vi "DC Attenuation Unflatten Test Parameters.vi"(9 "error in (no error)":errorcluster, 10 "Parameter String":string) -> (1 "error out":errorcluster, 2 "DC Attenuation Test Parameters":T2={"Stimulus"={"Use Instrument"=FALSE, "Normalize"=FALSE, "Blank Screen"=FALSE, "Measurement Type"=enum."Diode", "Range"=enum."Auto", "Resolution"=enum."Auto"}, "Measurement"={"Topology"=enum."PI-Network", "Lock Topology"=FALSE, "ATTN Calc"=enum."Power", "Zo"=50.0}, "Limits"=[], "Normalization"={"Normalized?"=FALSE, "Rab Value"=0.0, "Rac Value"=0.0, "Rbc Value"=0.0}}, 5 "Test Version":string)   [LabVIEW 2011]
uses:
  TypeDefs/DCA Test Parameters.ctl
  TypeDefs/DCA Stimulus Parameters.ctl
  TypeDefs/DCA Measurement Cluster.ctl
  TypeDefs/DCA Topology.ctl
  TypeDefs/DCA Attenuation Calculation.ctl
  TypeDefs/DCA Limit.ctl
  TypeDefs/DCA Limit Quantity.ctl
  TypeDefs/DCA Limit Comparison.ctl
  TypeDefs/DCA Limit Operation.ctl
  Test Referential Limit.ctl
  TypeDefs/DCA Calibration State.ctl
  Test Return Parameter.ctl
  TypeDefs/DCA Test Parameters v1.0-1.1.ctl
  TypeDefs/DCA Test Parameters v1.2.ctl
  TypeDefs/DCA Test Parameters v1.3-1.4.ctl
  TypeDefs/DCA Test Parameters v1.5.ctl
  TypeDefs/DCA Test Parameters v1.6-1.7.ctl
  TypeDefs/DCA Test Parameters v1.8.ctl
  TypeDefs/DCA Test Parameters v1.9.ctl
panel:
  in  "Return Parameter":T1
  out "Parameter Variant":variant
  in  "Required Instruments":string[](array[string])=["DMM", "SWI"]
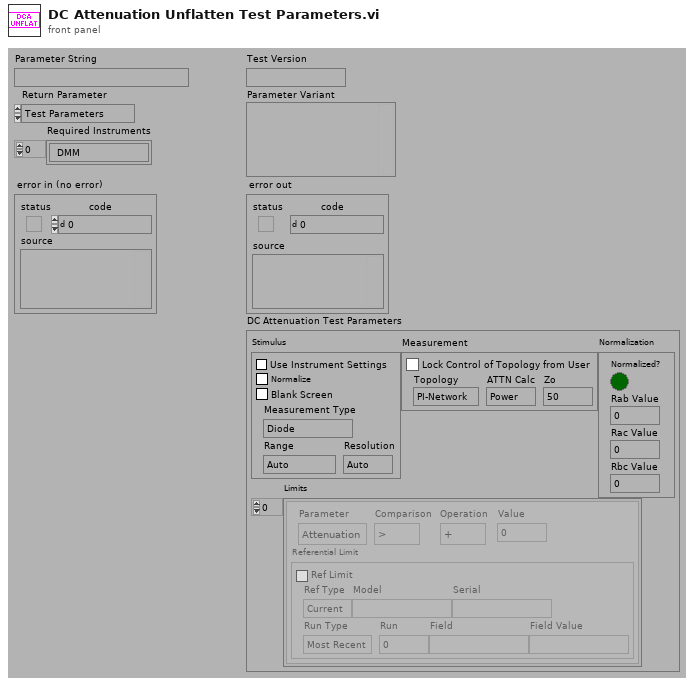
[diagram p1: front panel]
types:
  T1 = typedef "Test Return Parameter.ctl" = enum16{"Test Parameters", "Required Instruments", "Datasheets", "QuickMode"}
  T2 = typedef "DCA Test Parameters.ctl" = cluster{"Stimulus":T3, "Measurement":T4, "Limits":T7[], "Normalization":T12}
  T3 = typedef "DCA Stimulus Parameters.ctl" = cluster{"Use Instrument":bool, "Normalize":bool, "Blank Screen":bool, "Measurement Type":enum16{"Voltage DC", "Voltage DC Ratio", "Voltage AC", "Current DC", "Current AC", "Resistance", "Fresistance", "Frequency", "Period", "Continuity", "Diode"}, "Range":enum16{"Auto", "Minimum", "Maximum", "100", "1,000", "10,000", "100,000", "1,000,000", "10,000,000", "100,000,000"}, "Resolution":enum16{"Auto", "4 1/2", "5 1/2", "6 1/2"}}
  T4 = typedef "DCA Measurement Cluster.ctl" = cluster{"Topology":T5, "Lock Topology":bool, "ATTN Calc":T6, "Zo":dbl}
  T5 = typedef "DCA Topology.ctl" = enum32{"PI-Network", "T-Network"}
  T6 = typedef "DCA Attenuation Calculation.ctl" = enum32{"Power", "Voltage"}
  T7 = typedef "DCA Limit.ctl" = cluster{"Parameter":T8, "Comparison":T9, "Operation":T10, "Value":dbl, "Referential Limit":T11}
  T8 = typedef "DCA Limit Quantity.ctl" = enum16{"Attenuation", "Zin", "Zout", "R1", "R2", "R3", "Rab", "Rac", "Rbc"}
  T9 = typedef "DCA Limit Comparison.ctl" = enum16{">", ">=", "<", "<="}
  T10 = typedef "DCA Limit Operation.ctl" = enum16{"+", "-"}
  T11 = typedef "Test Referential Limit.ctl" = cluster{"Ref Limit":bool, "Ref Type":enum16{"Current", "Specify"}, "Model":string, "Serial":string, "Run Type":enum16{"Most Recent", "Run #", "Match Field"}, "Run":i32, "Field":string, "Field Value":string}
  T12 = typedef "DCA Calibration State.ctl" = cluster{"Normalized?":bool, "Rab Value":dbl, "Rac Value":dbl, "Rbc Value":dbl}
  T13 = typedef "DCA Test Parameters v1.0-1.1.ctl" = cluster{"Tag":string, "Use Instrument":bool, "Quick Mode":bool, "Topology":enum32{"Pi", "T"}, "Zo":dbl, "Range":u16, "Resolution":u16, "Blank Screen":bool, "Limits":cluster{"Quantity":enum16{"Attenuation", "Zin", "Zout", "R1", "R2", "R3", "Rab", "Rac", "Rbc"}, "Comparison":enum16{">", ">=", "<", "<="}, "Value":dbl}[], "Reports":i32[], "Lock Topology":bool}
  T14 = typedef "DCA Test Parameters v1.2.ctl" = cluster{"Tag":string, "Use Instrument":bool, "Quick Mode":bool, "Topology":enum32{"Pi", "T"}, "Zo":dbl, "Range":u16, "Resolution":u16, "Blank Screen":bool, "Limits":cluster{"Quantity":enum16{"Attenuation", "Zin", "Zout", "R1", "R2", "R3", "Rab", "Rac", "Rbc"}, "Comparison":enum16{">", ">=", "<", "<="}, "Value":dbl}[], "Reports":cluster{"Reports to Generate":i32[], "Print Reports":bool}, "Lock Topology":bool}
  T15 = typedef "DCA Test Parameters v1.3-1.4.ctl" = cluster{"Tag":string, "Use Instrument":bool, "Quick Mode":bool, "Topology":enum32{"Pi", "T"}, "Zo":dbl, "Range":u16, "Resolution":u16, "Blank Screen":bool, "Limits":cluster{"Quantity":enum16{"Attenuation", "Zin", "Zout", "R1", "R2", "R3", "Rab", "Rac", "Rbc"}, "Comparison":enum16{">", ">=", "<", "<="}, "Value":dbl}[], "Reports":cluster{"Reports to Generate":i32[], "Print Reports":bool}, "Lock Topology":bool, "Normalize":bool}
  T16 = typedef "DCA Test Parameters v1.5.ctl" = cluster{"Tag":string, "Use Instrument":bool, "Quick Mode":bool, "Topology":enum32{"Pi", "T"}, "Zo":dbl, "Range":u16, "Resolution":u16, "Blank Screen":bool, "Limits":cluster{"Quantity":enum16{"Attenuation", "Zin", "Zout", "R1", "R2", "R3", "Rab", "Rac", "Rbc"}, "Comparison":enum16{">", ">=", "<", "<=", "+", "-"}, "Value":dbl}[], "Reports":cluster{"Reports to Generate":i32[], "Print Reports":bool}, "Lock Topology":bool, "Normalize":bool, "ATTN Calc":enum32{"Power", "Voltage"}}
  T17 = typedef "DCA Test Parameters v1.6-1.7.ctl" = cluster{"Tag":string, "Use Instrument":bool, "Quick Mode":bool, "Topology":enum32{"Pi", "T"}, "Zo":dbl, "Range":u16, "Resolution":u16, "Blank Screen":bool, "Limits":cluster{"Quantity":enum16{"Attenuation", "Zin", "Zout", "R1", "R2", "R3", "Rab", "Rac", "Rbc"}, "Comparison":enum16{">", ">=", "<", "<=", "+", "-"}, "Operation":enum16{"+", "-"}, "Value":dbl, "Ref Limit":bool, "Ref Type":enum32{"Current", "Specify"}, "Model":string, "Serial":string, "Run Type":enum32{"Most Recent", "Run #"}, "Run":i32, "Match Property":bool, "Property":string, "Property Value":string}[], "Reports":cluster{"Reports to Generate":i32[], "Print Reports":bool}, "Lock Topology":bool, "Normalize":bool, "ATTN Calc":enum32{"Power", "Voltage"}}
  T18 = typedef "DCA Test Parameters v1.8.ctl" = cluster{"Tag":string, "Use Instrument":bool, "Quick Mode":bool, "Topology":enum32{"Pi", "T"}, "Zo":dbl, "Range":u16, "Resolution":u16, "Blank Screen":bool, "Limits":cluster{"Quantity":enum16{"Attenuation", "Zin", "Zout", "R1", "R2", "R3", "Rab", "Rac", "Rbc"}, "Comparison":enum16{">", ">=", "<", "<=", "+", "-"}, "Operation":enum16{"+", "-"}, "Value":dbl, "Ref Limit":bool, "Ref Type":enum32{"Current", "Specify"}, "Model":string, "Serial":string, "Run Type":enum32{"Most Recent", "Run #"}, "Run":i32, "Match Property":bool, "Property":string, "Property Value":string}[], "Datasheets":cluster{"Datasheets to Generate":i32[], "Print Datasheets":bool}, "Lock Topology":bool, "Normalize":bool, "ATTN Calc":enum32{"Power", "Voltage"}}
  T19 = typedef "DCA Test Parameters v1.9.ctl" = cluster{"Stimulus":cluster{"Use Instrument":bool, "Normalize":bool, "Blank Screen":bool, "Measurement Type":enum16{"Voltage DC", "Voltage DC Ratio", "Voltage AC", "Current DC", "Current AC", "Resistance", "Fresistance", "Frequency", "Period", "Continuity", "Diode"}, "Range":enum16{"Auto", "Minimum", "Maximum", "100", "1,000", "10,000", "100,000", "1,000,000", "10,000,000", "100,000,000"}, "Resolution":enum16{"Auto", "4 1/2", "5 1/2", "6 1/2"}}, "Measurement":cluster{"Topology":enum32{"PI-Network", "T-Network"}, "Lock Topology":bool, "ATTN Calc":enum32{"Power", "Voltage"}, "Zo":dbl}, "Limits":cluster{"Parameter":enum16{"Attenuation", "Zin", "Zout", "R1", "R2", "R3", "Rab", "Rac", "Rbc"}, "Comparison":enum16{">", ">=", "<", "<="}, "Operation":enum16{"+", "-"}, "Value":dbl, "Referential Limit":cluster{"Ref Limit":bool, "Ref Type":enum16{"Current", "Specify"}, "Model":string, "Serial":string, "Run Type":enum16{"Most Recent", "Run #", "Match Field"}, "Run":i32, "Field":string, "Field Value":string}}[], "Datasheets":cluster{"Datasheet to Generate":i32, "Print Datasheets":bool}[]}
  T20 = typedef "Test Datasheets v1.0-4.0.ctl" = cluster{"Datasheet to Generate":i32, "Print Datasheets":bool}[]
  T21 = typedef "DCA Test Parameters v1.10-1.11.ctl" = cluster{"Stimulus":T3, "Measurement":T4, "Limits":T7[]}
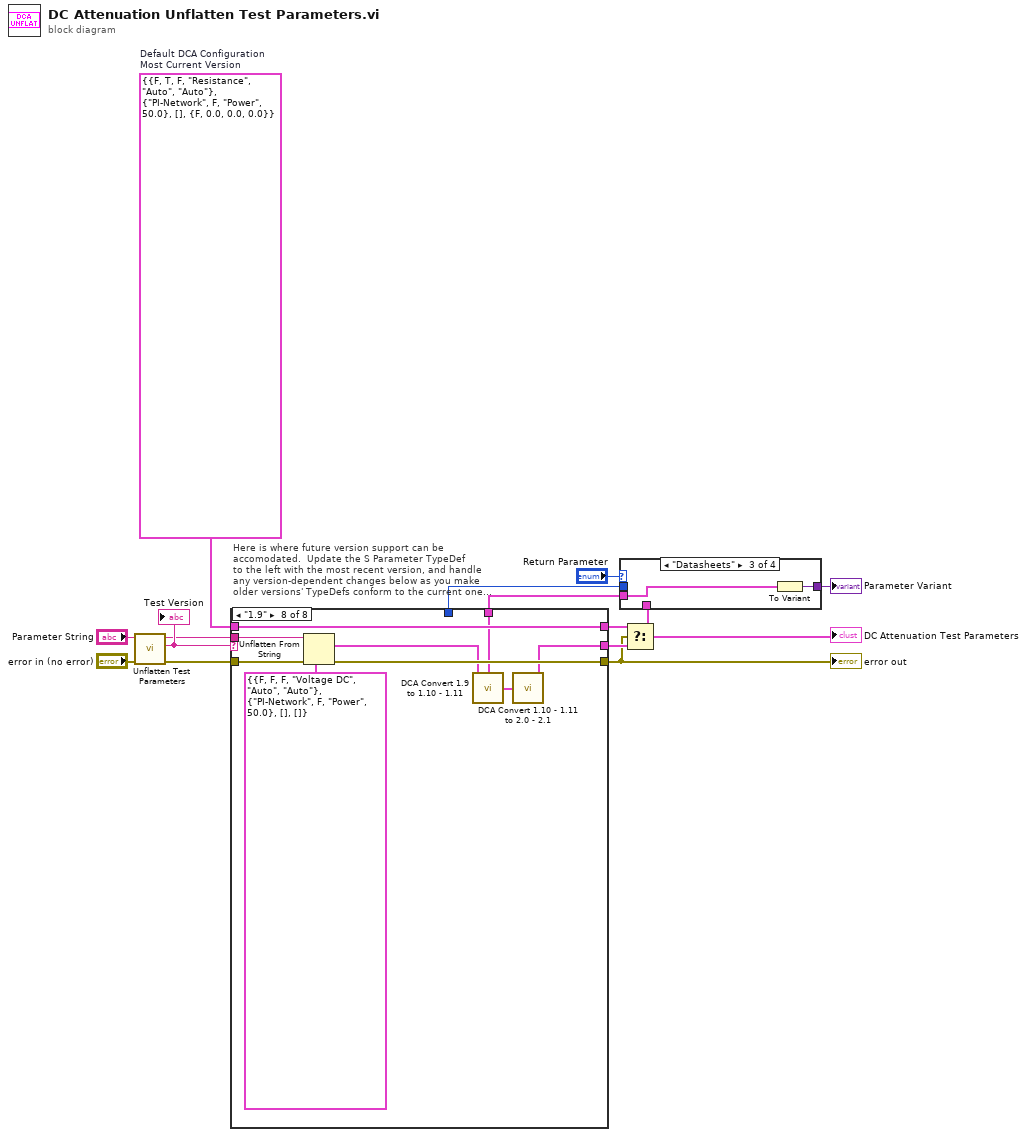
[diagram p0: block diagram]
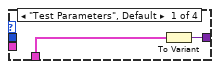
[diagram p2: hidden frame]
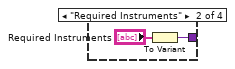
[diagram p3: hidden frame]
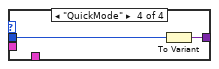
[diagram p4: hidden frame]
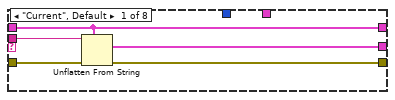
[diagram p5: hidden frame]
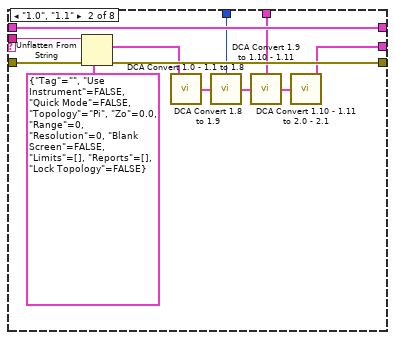
[diagram p6: hidden frame]
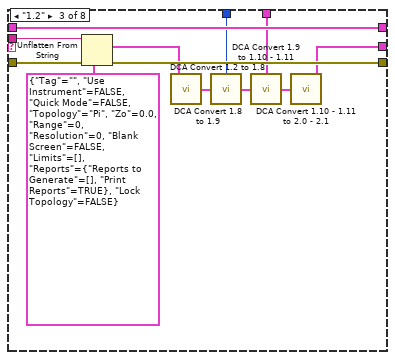
[diagram p7: hidden frame]
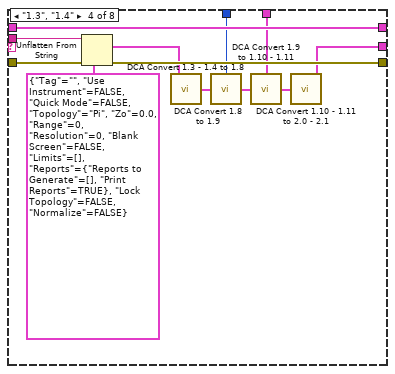
[diagram p8: hidden frame]
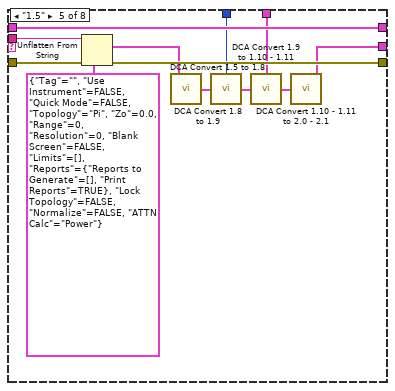
[diagram p9: hidden frame]
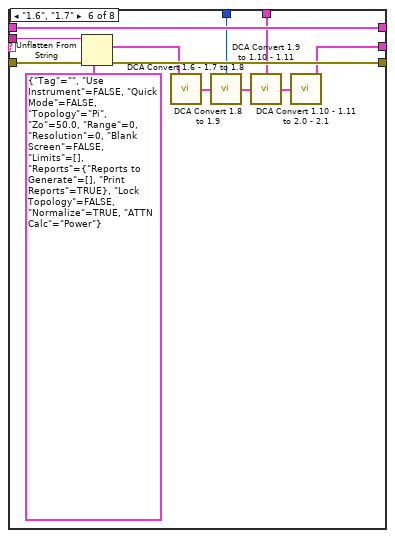
[diagram p10: hidden frame]
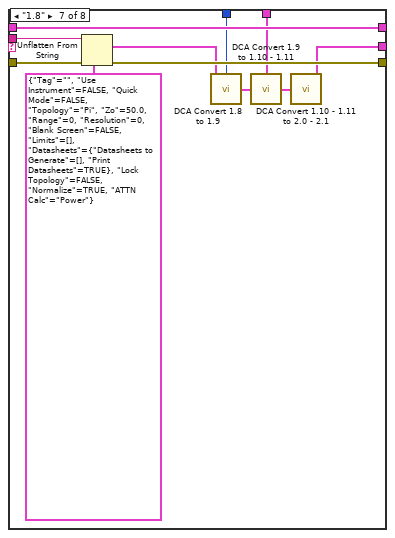
[diagram p11: hidden frame]
diagram:
  w4 = T2 {"Stimulus"={"Use Instrument"=FALSE, "Normalize"=TRUE, "Blank Screen"=FALSE, "Measurement Type"=enum."Resistance", "Range"=enum."Auto", "Resolution"=enum."Auto"}, "Measurement"={"Topology"=enum."PI-Network", "Lock Topology"=FALSE, "ATTN Calc"=enum."Power", "Zo"=50.0}, "Limits"=[], "Normalization"={"Normalized?"=FALSE, "Rab Value"=0.0, "Rac Value"=0.0, "Rbc Value"=0.0}}  # Default DCA Configuration Most Current Version
  # "Here is where future version support can be\naccomodated.  Update the S Parameter TypeDef\nto the left with the most recent version, and handle\nany version-dependent changes below as you make\nolder versions' TypeDefs conform to the current one..."
  n1 = call "Unflatten Test Parameters.vi"("error in (no error)"="error in (no error)", "Flattened Test Parameters with Version (\"\")"="Parameter String") -> ("error out"=w5:errorcluster, "Test Version"=w13:string, "Flat Test Parameters"=w12:string)  [unwired: 3 out]
  "Test Version" <- w13
  n2 = case shown="\"1.9\"" w13 {
    tunnel: [w18 w20 w32 w44 w56 w68 w80 w91] -> w11
    tunnel: w12 -> [w19 w31 w43 w55 w67 w79 w90 w99]
    tunnel: [w16 w28 w40 w51 w65 w78 w89 w98] -> w6
    tunnel: w5 -> [w17 w29 w41 w52 w64 w77 w88 w97]
    tunnel: w4 -> [w15 w27 w39 w53 w63 w76 w87 w96]
    tunnel: [w15 w27 w39 w53 w63 w76 w87 w96] -> w3
    tunnel: [_ w24 w36 w48 w60 w72 w84 _] -> w2
    tunnel: [_ w23 w34 w47 w59 w71 w82 w93] -> w1
    frame "Current", Default {
      n3 = Unflatten From String(type=w15, binary string=w19, error in (no error)=w17) -> (value=w18:T2, error out=w16:errorcluster)  [unwired: 3 out]
    }
    frame "1.0", "1.1" {
      n4 = Unflatten From String(type=T13 {"Tag"="", "Use Instrument"=FALSE, "Quick Mode"=FALSE, "Topology"=enum."Pi", "Zo"=0.0, "Range"=0, "Resolution"=0, "Blank Screen"=FALSE, "Limits"=[], "Reports"=[], "Lock Topology"=FALSE} ("DCA Test Parameters"), binary string=w31, error in (no error)=w29) -> (value=w26:T13, error out=w28:errorcluster)  [unwired: 3 out]
      n5 = call "DCA Convert 1.0 - 1.1 to 1.8.vi"("DCA 1.0 - 1.1 Test Parameters"=w26) -> ("DCA 1.8 Test Parameters"=w25:T18)
      n6 = call "DCA Convert 1.8 to 1.9.vi"("DCA 1.8 Test Parameters"=w25) -> ("QuickMode"=w24:i8, "DCA 1.9 Test Parameters"=w22:T19)
      n7 = call "DCA Convert 1.9 to 1.10 - 1.11.vi"("DCA 1.9 Test Parameters"=w22) -> ("Datasheets"=w23:T20, "DCA 1.10 - 1.11 Test Parameters"=w21:T21)
      n8 = call "DCA Convert 1.10 - 1.11 to 2.0 - 2.1.vi"("DCA 1.10 - 1.11 Test Parameters"=w21) -> ("DCA 2.0 - 2.1 Test Parameters"=w20:T2)  [unwired: 1 out]
    }
    frame "1.2" {
      n9 = Unflatten From String(type=T14 {"Tag"="", "Use Instrument"=FALSE, "Quick Mode"=FALSE, "Topology"=enum."Pi", "Zo"=0.0, "Range"=0, "Resolution"=0, "Blank Screen"=FALSE, "Limits"=[], "Reports"={"Reports to Generate"=[], "Print Reports"=TRUE}, "Lock Topology"=FALSE} ("DCA Test Parameters"), binary string=w43, error in (no error)=w41) -> (value=w37:T14, error out=w40:errorcluster)  [unwired: 3 out]
      n10 = call "DCA Convert 1.2 to 1.8.vi"("DCA 1.2 Test Parameters"=w37) -> ("DCA 1.8 Test Parameters"=w38:T18)
      n11 = call "DCA Convert 1.8 to 1.9.vi"("DCA 1.8 Test Parameters"=w38) -> ("QuickMode"=w36:i8, "DCA 1.9 Test Parameters"=w35:T19)
      n12 = call "DCA Convert 1.9 to 1.10 - 1.11.vi"("DCA 1.9 Test Parameters"=w35) -> ("Datasheets"=w34:T20, "DCA 1.10 - 1.11 Test Parameters"=w33:T21)
      n13 = call "DCA Convert 1.10 - 1.11 to 2.0 - 2.1.vi"("DCA 1.10 - 1.11 Test Parameters"=w33) -> ("DCA 2.0 - 2.1 Test Parameters"=w32:T2)  [unwired: 1 out]
    }
    frame "1.3", "1.4" {
      n14 = Unflatten From String(type=T15 {"Tag"="", "Use Instrument"=FALSE, "Quick Mode"=FALSE, "Topology"=enum."Pi", "Zo"=0.0, "Range"=0, "Resolution"=0, "Blank Screen"=FALSE, "Limits"=[], "Reports"={"Reports to Generate"=[], "Print Reports"=TRUE}, "Lock Topology"=FALSE, "Normalize"=FALSE} ("DCA Test Parameters"), binary string=w55, error in (no error)=w52) -> (value=w50:T15, error out=w51:errorcluster)  [unwired: 3 out]
      n15 = call "DCA Convert 1.3 - 1.4 to 1.8.vi"("DCA 1.3 - 1.4 Test Parameters"=w50) -> ("DCA 1.8 Test Parameters"=w49:T18)
      n16 = call "DCA Convert 1.8 to 1.9.vi"("DCA 1.8 Test Parameters"=w49) -> ("QuickMode"=w48:i8, "DCA 1.9 Test Parameters"=w46:T19)
      n17 = call "DCA Convert 1.9 to 1.10 - 1.11.vi"("DCA 1.9 Test Parameters"=w46) -> ("Datasheets"=w47:T20, "DCA 1.10 - 1.11 Test Parameters"=w45:T21)
      n18 = call "DCA Convert 1.10 - 1.11 to 2.0 - 2.1.vi"("DCA 1.10 - 1.11 Test Parameters"=w45) -> ("DCA 2.0 - 2.1 Test Parameters"=w44:T2)  [unwired: 1 out]
    }
    frame "1.5" {
      n19 = Unflatten From String(type=T16 {"Tag"="", "Use Instrument"=FALSE, "Quick Mode"=FALSE, "Topology"=enum."Pi", "Zo"=0.0, "Range"=0, "Resolution"=0, "Blank Screen"=FALSE, "Limits"=[], "Reports"={"Reports to Generate"=[], "Print Reports"=TRUE}, "Lock Topology"=FALSE, "Normalize"=FALSE, "ATTN Calc"=enum."Power"} ("DCA Test Parameters"), binary string=w67, error in (no error)=w64) -> (value=w62:T16, error out=w65:errorcluster)  [unwired: 3 out]
      n20 = call "DCA Convert 1.5 to 1.8.vi"("DCA 1.5 Test Parameters"=w62) -> ("DCA 1.8 Test Parameters"=w61:T18)
      n21 = call "DCA Convert 1.8 to 1.9.vi"("DCA 1.8 Test Parameters"=w61) -> ("QuickMode"=w60:i8, "DCA 1.9 Test Parameters"=w58:T19)
      n22 = call "DCA Convert 1.9 to 1.10 - 1.11.vi"("DCA 1.9 Test Parameters"=w58) -> ("Datasheets"=w59:T20, "DCA 1.10 - 1.11 Test Parameters"=w57:T21)
      n23 = call "DCA Convert 1.10 - 1.11 to 2.0 - 2.1.vi"("DCA 1.10 - 1.11 Test Parameters"=w57) -> ("DCA 2.0 - 2.1 Test Parameters"=w56:T2)  [unwired: 1 out]
    }
    frame "1.6", "1.7" {
      n24 = Unflatten From String(type=T17 {"Tag"="", "Use Instrument"=FALSE, "Quick Mode"=FALSE, "Topology"=enum."Pi", "Zo"=50.0, "Range"=0, "Resolution"=0, "Blank Screen"=FALSE, "Limits"=[], "Reports"={"Reports to Generate"=[], "Print Reports"=TRUE}, "Lock Topology"=FALSE, "Normalize"=TRUE, "ATTN Calc"=enum."Power"} ("DCA Test Parameters"), binary string=w79, error in (no error)=w77) -> (value=w74:T17, error out=w78:errorcluster)  [unwired: 3 out]
      n25 = call "DCA Convert 1.6 - 1.7 to 1.8.vi"("DCA 1.6 - 1.7 Test Parameters"=w74) -> ("DCA 1.8 Test Parameters"=w73:T18)
      n26 = call "DCA Convert 1.8 to 1.9.vi"("DCA 1.8 Test Parameters"=w73) -> ("QuickMode"=w72:i8, "DCA 1.9 Test Parameters"=w70:T19)
      n27 = call "DCA Convert 1.9 to 1.10 - 1.11.vi"("DCA 1.9 Test Parameters"=w70) -> ("Datasheets"=w71:T20, "DCA 1.10 - 1.11 Test Parameters"=w69:T21)
      n28 = call "DCA Convert 1.10 - 1.11 to 2.0 - 2.1.vi"("DCA 1.10 - 1.11 Test Parameters"=w69) -> ("DCA 2.0 - 2.1 Test Parameters"=w68:T2)  [unwired: 1 out]
    }
    frame "1.8" {
      n29 = Unflatten From String(type=T18 {"Tag"="", "Use Instrument"=FALSE, "Quick Mode"=FALSE, "Topology"=enum."Pi", "Zo"=50.0, "Range"=0, "Resolution"=0, "Blank Screen"=FALSE, "Limits"=[], "Datasheets"={"Datasheets to Generate"=[], "Print Datasheets"=TRUE}, "Lock Topology"=FALSE, "Normalize"=TRUE, "ATTN Calc"=enum."Power"} ("DCA Test Parameters"), binary string=w90, error in (no error)=w88) -> (value=w85:T18, error out=w89:errorcluster)  [unwired: 3 out]
      n30 = call "DCA Convert 1.8 to 1.9.vi"("DCA 1.8 Test Parameters"=w85) -> ("QuickMode"=w84:i8, "DCA 1.9 Test Parameters"=w83:T19)
      n31 = call "DCA Convert 1.9 to 1.10 - 1.11.vi"("DCA 1.9 Test Parameters"=w83) -> ("Datasheets"=w82:T20, "DCA 1.10 - 1.11 Test Parameters"=w81:T21)
      n32 = call "DCA Convert 1.10 - 1.11 to 2.0 - 2.1.vi"("DCA 1.10 - 1.11 Test Parameters"=w81) -> ("DCA 2.0 - 2.1 Test Parameters"=w80:T2)  [unwired: 1 out]
    }
    frame "1.9" {
      n33 = Unflatten From String(type=T19 {"Stimulus"={"Use Instrument"=FALSE, "Normalize"=FALSE, "Blank Screen"=FALSE, "Measurement Type"=enum."Voltage DC", "Range"=enum."Auto", "Resolution"=enum."Auto"}, "Measurement"={"Topology"=enum."PI-Network", "Lock Topology"=FALSE, "ATTN Calc"=enum."Power", "Zo"=50.0}, "Limits"=[], "Datasheets"=[]} ("DCA Test Parameters"), binary string=w99, error in (no error)=w97) -> (value=w94:T19, error out=w98:errorcluster)  [unwired: 3 out]
      n34 = call "DCA Convert 1.9 to 1.10 - 1.11.vi"("DCA 1.9 Test Parameters"=w94) -> ("Datasheets"=w93:T20, "DCA 1.10 - 1.11 Test Parameters"=w92:T21)
      n35 = call "DCA Convert 1.10 - 1.11 to 2.0 - 2.1.vi"("DCA 1.10 - 1.11 Test Parameters"=w92) -> ("DCA 2.0 - 2.1 Test Parameters"=w91:T2)  [unwired: 1 out]
    }
  }
  "error out" <- w6
  n36 = Select(t=w3, s=w6, f=w11) -> (s? t:f=w8:T2)
  "DC Attenuation Test Parameters" <- w8
  n37 = case shown="\"Datasheets\"" "Return Parameter" {
    tunnel: [w101 w103 w105 w107] -> w9
    tunnel: w8 -> [w100 _ _ _]
    tunnel: w2 -> [_ _ _ w106]
    tunnel: w1 -> [_ _ w104 _]
    frame "Test Parameters", Default {
      n38 = To Variant(anything=w100) -> (Variant=w101:variant)
    }
    frame "Required Instruments" {
      n39 = To Variant(anything="Required Instruments") -> (Variant=w103:variant)
    }
    frame "Datasheets" {
      n40 = To Variant(anything=w104) -> (Variant=w105:variant)
    }
    frame "QuickMode" {
      n41 = To Variant(anything=w106) -> (Variant=w107:variant)
    }
  }
  "Parameter Variant" <- w9
